vi "PD4-C Front Panel.vi"() -> ()   [LabVIEW 2021]
uses:
  Old and Failed/Nanotec_PDC-4 Lib/Nanotech PDC-4.lvlib
panel:
  in  "Write":T1={"Data (dec)"=0, FALSE, "Index"="``", "Sub-Index"="\u0000", "Data-Size (in Byte)"=1} {"Data-Size (in Byte)" min=1 max=4 step=1 format="%x"; "Data (dec)" step=1}
  out "error out":errorcluster
  out "Torque Nm":i32
  out "Motor Running":bool
  out "Closed Loop Available":bool
  out "Torque / Current\n%":i32
  out "Motor Current Max\nmA":i32
  out "rpm":dbl(knob) scale=0.0..10.0
  in  "Stop Program":bool
  in  "Speed\n rpm":dbl(knob) scale=0.0..10.0
  in  "Reverse Button":bool
  in  "Forward Button":bool
  in  "Stop Button":bool
  in  "Start Button":bool
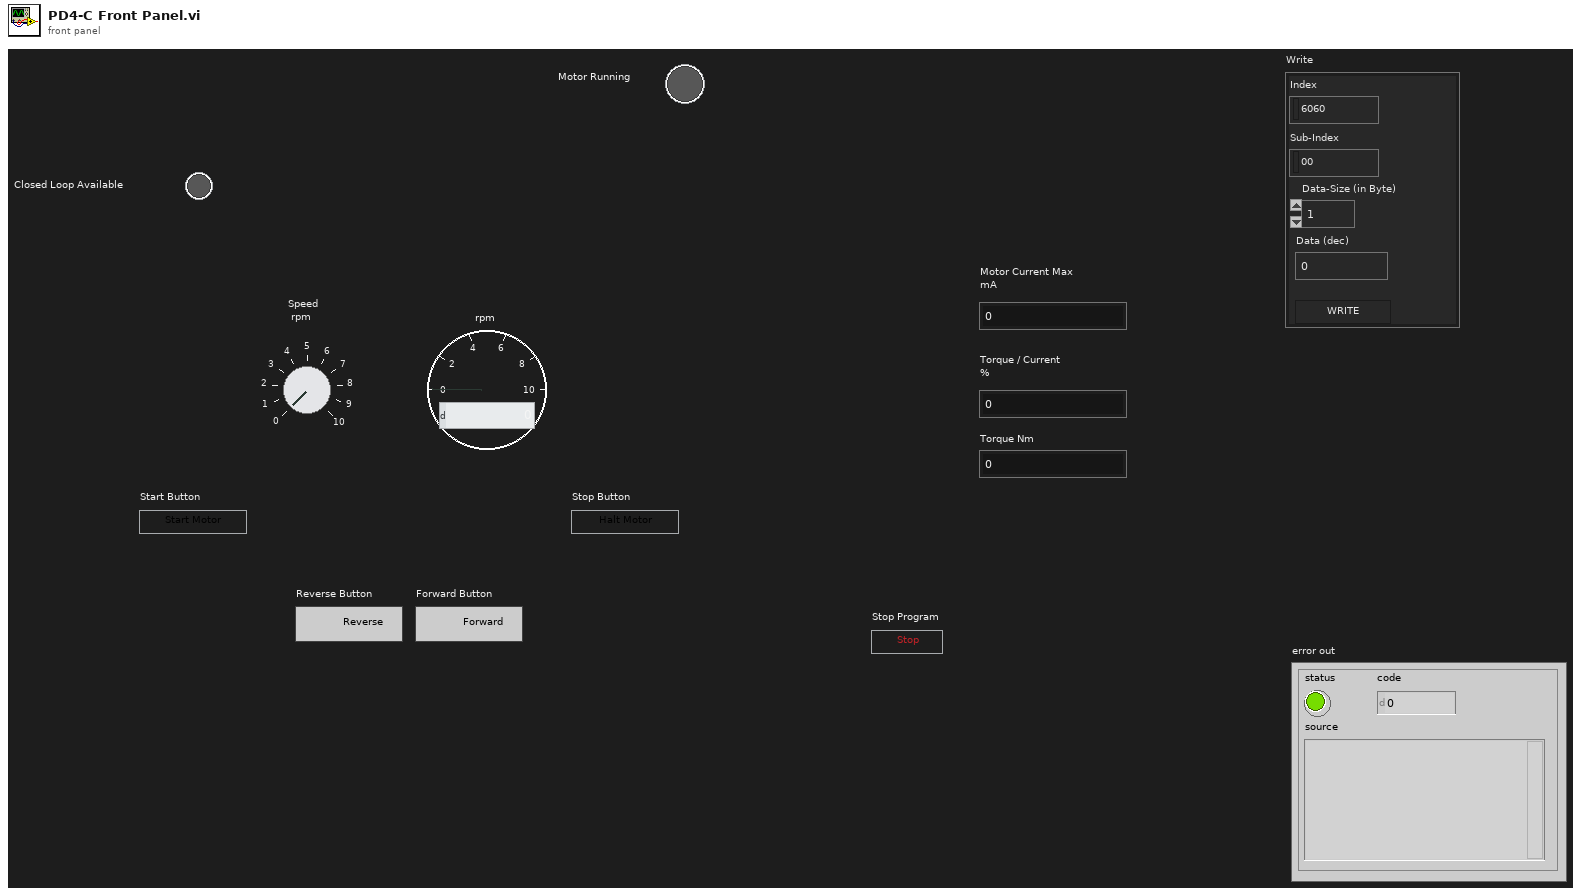
[diagram p1: front panel]
types:
  T1 = cluster{"Data (dec)":i32, bool, "Index":string, "Sub-Index":string, "Data-Size (in Byte)":u8}
  T2 = cluster{"Data (dec)":i32, "write":bool, "Index":string, "Sub-Index":string, "Data-Size (in Byte)":u8}
  T3 = cluster{"Index":string, "Sub-Index":string, "Data-Size (in Byte)":u8}
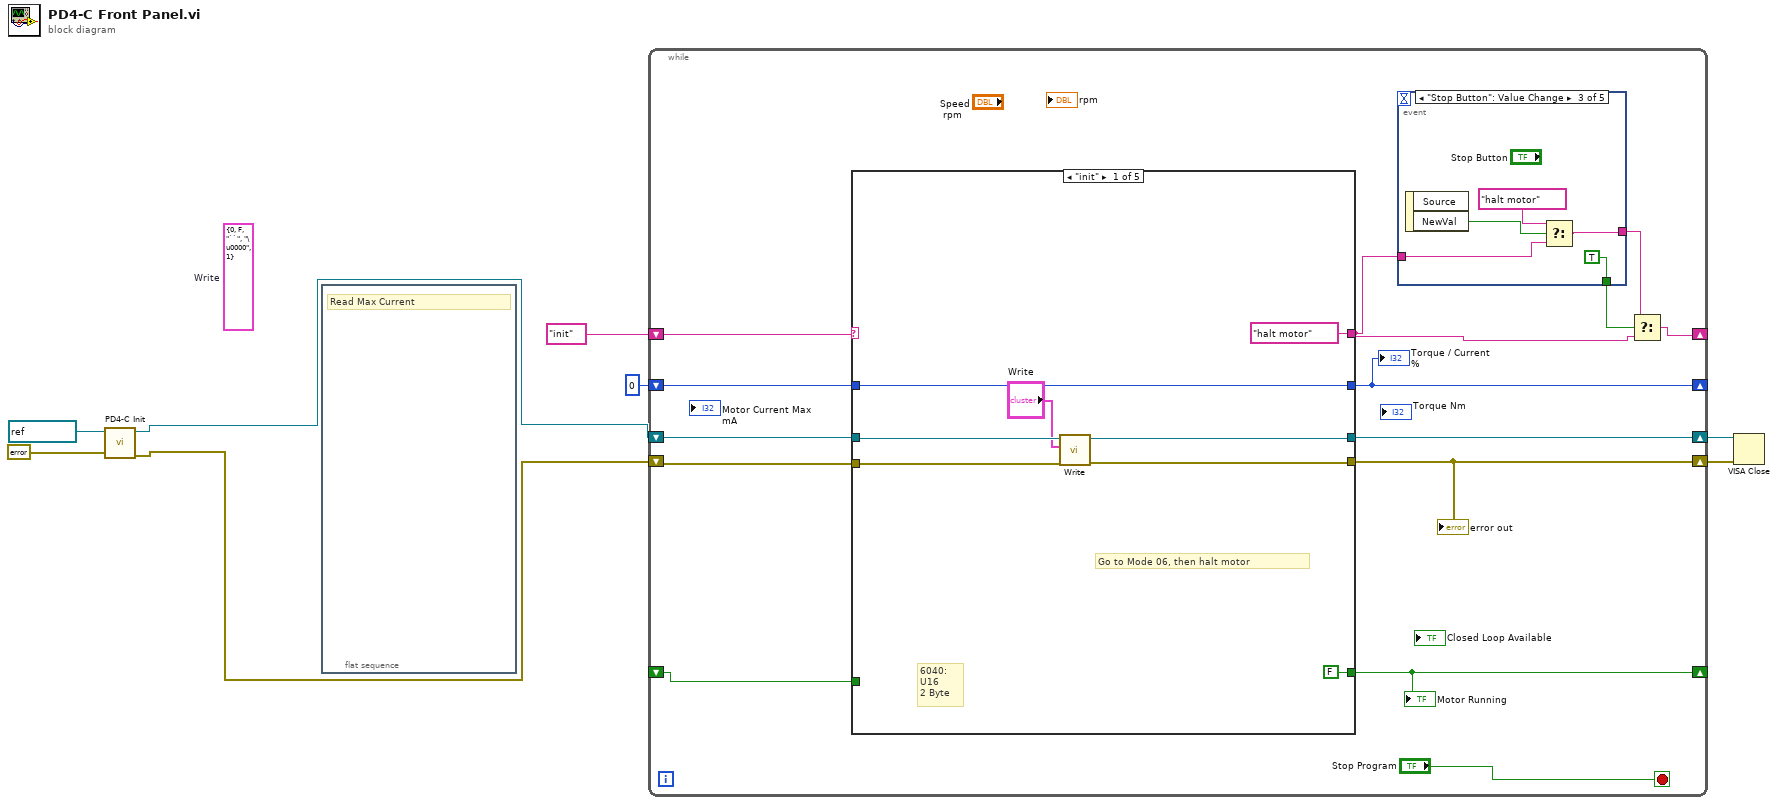
[diagram p0: block diagram]
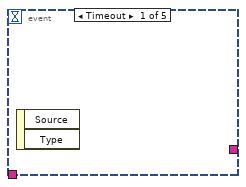
[diagram p2: hidden frame]
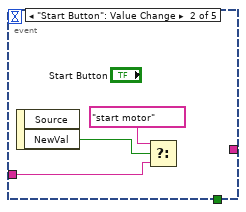
[diagram p3: hidden frame]
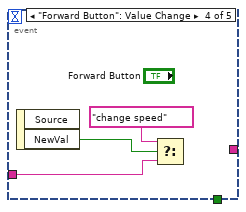
[diagram p4: hidden frame]
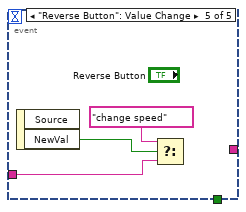
[diagram p5: hidden frame]
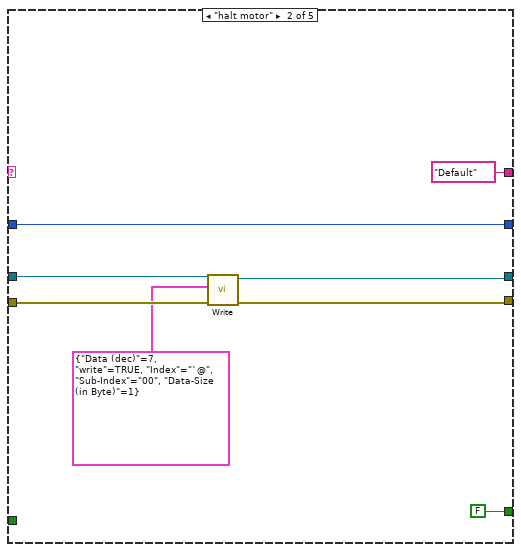
[diagram p6: hidden frame]
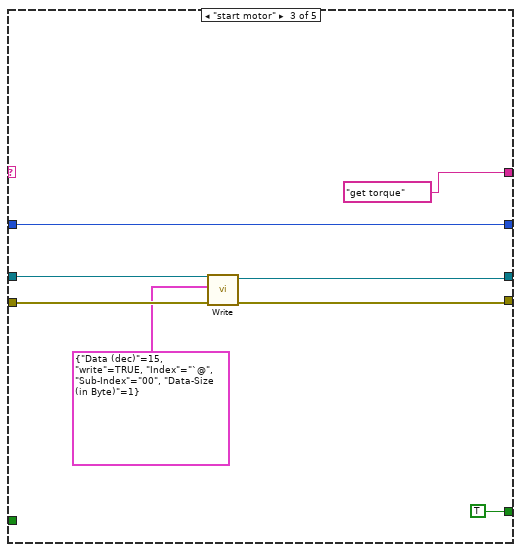
[diagram p7: hidden frame]
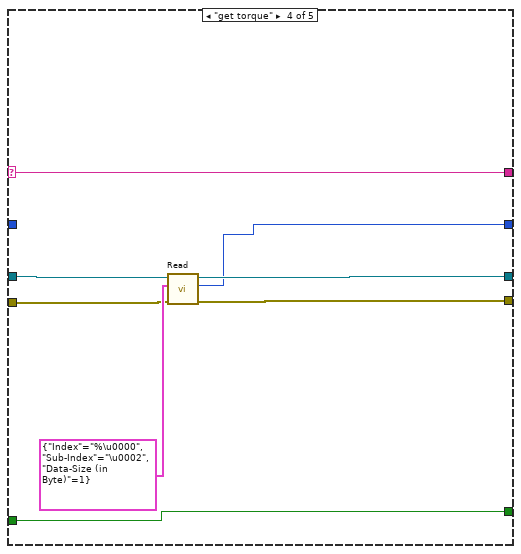
[diagram p8: hidden frame]
diagram:
  (unwired) T1 {"Data (dec)"=0, FALSE, "Index"="``", "Sub-Index"="\u0000", "Data-Size (in Byte)"=1}  # Write
  n1 = call "PD4-C Init.vi"("error in (no error)"=errorcluster {"status"=FALSE, "code"=0, "source"=""}, "VISA Refnum in"=refnum<visa-resource-name> "COM15") -> ("error out"=w1:errorcluster, "VISA Refnum out"=w2:refnum<visa-resource-name>)  [unwired: 8 in]
  n2 = flat-sequence {
    frame #0 {
      # "Read Max Current"
    }
  }
  n3 = while {
    shift-right: [w21] -> w6
    shift-left: w2 -> [w22]
    shift-right: [w20] -> w7
    shift-left: w1 -> [w17]
    shift-right: [w9] -> _
    shift-left: "init" -> [w19]
    shift-right: [w16] -> _
    shift-left: 0 ("Answer") -> [w15]
    shift-right: [w14] -> _
    shift-left: _ -> [w13]
    stop <- "Stop Program" stop-if-true
    n4 = case shown="\"init\"" w19 {
      selector: w19 -> [_ _ _ w63 w73]
      tunnel: w22 -> [w41 w52 w60 w66 w71]
      tunnel: [w39 w50 w58 w65 w71] -> w21
      tunnel: w17 -> [w40 w51 w59 w67 w70]
      tunnel: [w38 w49 w57 w64 w70] -> w20
      tunnel: [w43 w47 w55 w62 w72] -> w16
      tunnel: ["halt motor" "Default" "get torque" w63 w73] -> w11
      tunnel: w15 -> [w43 w47 w55 _ w72]
      tunnel: [FALSE ("Motor Running") FALSE ("Motor Running") TRUE ("Motor Running") w61 w69] -> w14
      tunnel: w13 -> [_ _ _ w61 w69]
      frame "init" {
        # "6040:\nU16\n2 Byte"
        # "Go to Mode 06, then halt motor"
        n5 = call "Write.vi"("error in"=w40, "Write"="Write", "ComPort In"=w41) -> ("error out"=w38:errorcluster, "ComPort Out"=w39:refnum<visa-resource-name>)  [unwired: 7 in]
      }
      frame "halt motor" {
        n6 = call "Write.vi"("error in"=w51, "Write"=T2 {"Data (dec)"=7, "write"=TRUE, "Index"="`@", "Sub-Index"="00", "Data-Size (in Byte)"=1}, "ComPort In"=w52) -> ("error out"=w49:errorcluster, "ComPort Out"=w50:refnum<visa-resource-name>)  [unwired: 7 in]
      }
      frame "start motor" {
        n7 = call "Write.vi"("error in"=w59, "Write"=T2 {"Data (dec)"=15, "write"=TRUE, "Index"="`@", "Sub-Index"="00", "Data-Size (in Byte)"=1}, "ComPort In"=w60) -> ("error out"=w57:errorcluster, "ComPort Out"=w58:refnum<visa-resource-name>)  [unwired: 7 in]
      }
      frame "get torque" {
        n8 = call "Read.vi"("error out"=w67, "Command"=T3 {"Index"="%\u0000", "Sub-Index"="\u0002", "Data-Size (in Byte)"=1}, "ComPort In"=w66) -> ("error out 2"=w64:errorcluster, "Answer"=w62:i32, "ComPort Out"=w65:refnum<visa-resource-name>)  [unwired: 6 in]
      }
      frame Default {
      }
    }
    "Torque / Current\n%" <- w16
    "Motor Running" <- w14
    "error out" <- w20
    n9 = event shown="[2] \"Stop Button\": Value Change" {
      selector: _ -> [_ _ _ _ _]
      dyn-events: _ -> [_ _ _ _ _]
      timeout: _ -> [_ _ _ _ _]
      tunnel: w11 -> [_ w24 w29 w32 w35]
      tunnel: [_ _ TRUE ("s") _ _] -> w12
      tunnel: [_ _ w26 _ _] -> w10
      event Timeout {
        n10 = event-data() -> ()  [unwired: 1 in, 2 out]
      }
      event "Start Button": Value Change {
        n11 = event-data() -> ("NewVal"=w23:bool)  [unwired: 1 in, 1 out]
        n12 = Select(t="start motor", s=w23, f=w24) -> ()  [unwired: 1 out]
      }
      event "Stop Button": Value Change {
        n13 = event-data() -> ("NewVal"=w28:bool)  [unwired: 1 in, 1 out]
        n14 = Select(t="halt motor", s=w28, f=w29) -> (s? t:f=w26:string)
      }
      event "Forward Button": Value Change {
        n15 = event-data() -> ("NewVal"=w31:bool)  [unwired: 1 in, 1 out]
        n16 = Select(t="change speed", s=w31, f=w32) -> ()  [unwired: 1 out]
      }
      event "Reverse Button": Value Change {
        n17 = event-data() -> ("NewVal"=w34:bool)  [unwired: 1 in, 1 out]
        n18 = Select(t="change speed", s=w34, f=w35) -> ()  [unwired: 1 out]
      }
    }
    n19 = Select(t=w10, s=w12, f=w11) -> (s? t:f=w9:string)
  }
  n20 = VISA Close(VISA resource name=w6, error in (no error)=w7) -> ()  [unwired: 1 out]
